vi "SubVi_timer.vi"(6 "stop":bool, 8 "Numeric 2":u32, 10 "Numeric":u32) -> (0 "Numeric 4":u32, 2 "Numeric 3":u32)   [LabVIEW 2024, in "Road.lvlib" / "GUI.lvlib"]
uses:
  GUI.lvlib
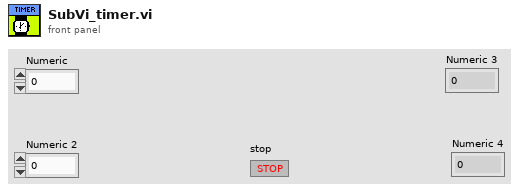
[diagram p1: front panel]
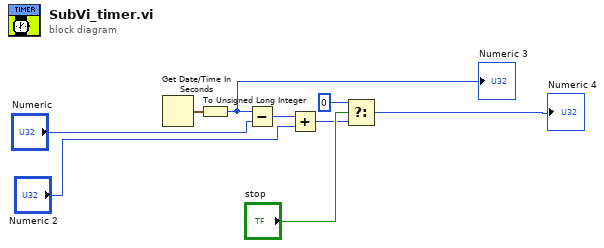
[diagram p0: block diagram]
diagram:
  n1 = Get Date/Time In Seconds() -> (seconds since 1Jan1904=w6:timestamp)
  n2 = To Unsigned Long Integer(number=w6) -> (unsigned 32bit integer=w4:u32)
  "Numeric 3" <- w4
  n3 = Subtract(x=w4, y="Numeric") -> (x-y=w7:u32)
  n4 = Add(x=w7, y="Numeric 2") -> (x+y=w8:u32)
  n5 = Select(t=u32 0, s="stop", f=w8) -> (s? t:f=→"Numeric 4":u32)
